vi "DigitalOscilloscope.vi"() -> ()   [LabVIEW 2014]
panel:
  out "error out":errorcluster
  in  "Digitalizing Parameters":T1
  out "Waveform Graph":dynamicdata(graph)
  in  "Stop":bool
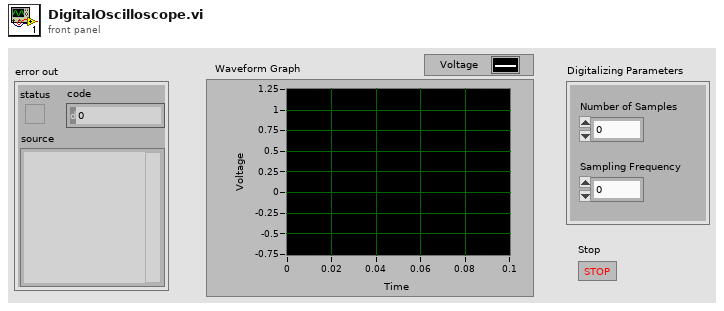
[diagram p1: front panel]
types:
  T1 = cluster{"Number of Samples":dbl, "Sampling Frequency":dbl}
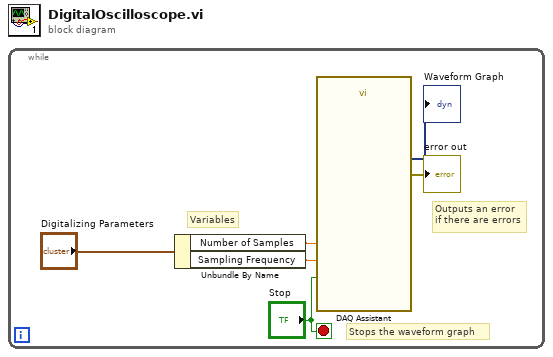
[diagram p0: block diagram]
diagram:
  n1 = while {
    stop <- "Stop" stop-if-true
    # "Outputs an error \nif there are errors"
    # "Stops the waveform graph"
    # "Variables"
    n2 = Unbundle By Name("Digitalizing Parameters") -> ("Number of Samples"=w6:dbl, "Sampling Frequency"=w5:dbl)
    n3 = call "DAQ Assistant"("rate"=w5, "number of samples"=w6, "stop (T)"="Stop") -> ("data"=→"Waveform Graph":dynamicdata, "error out"=→"error out":errorcluster)  [unwired: 14 in, 1 out]
  }
